vi "Build_Header_String_Array.vi"(0 "ERD Name Array In":string[](array[string]), 1 "ERD Number Array In":string[](array[string]), 2 "ERD Name List":string[](array[string])=[""], 3 "New Header?":bool, 4 "ERD Number":u16) -> (14 "ERD Name Array Out":string[](array[string]), 15 "ERD Number Array Out":string[](array[string]))   [LabVIEW 2021]
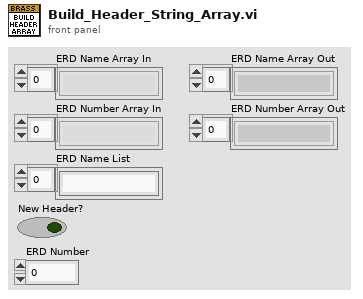
[diagram p1: front panel]
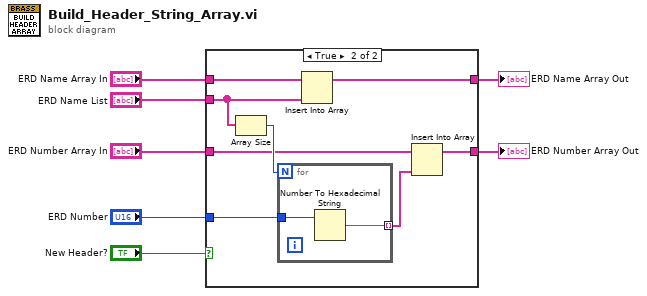
[diagram p0: block diagram]
diagram:
  n1 = case shown="True" "New Header?" {
    tunnel: "ERD Number Array In" -> [w9 w12]
    tunnel: "ERD Number" -> [_ w17]
    tunnel: [w9 w10] -> w4
    tunnel: "ERD Name Array In" -> [w8 w16]
    tunnel: "ERD Name List" -> [_ w13]
    tunnel: [w8 w15] -> w7
    frame False {
    }
    frame True {
      n2 = Array Size(array=w13) -> (size(s)=w14:i32)
      n3 = for {
        N: w14 -> [_]
        tunnel: w17 -> [w19]
        tunnel: [w18] -> w11 mode=indexing
        n4 = Number To Hexadecimal String(2:w19) -> (0:w18:string)  [unwired: 1 in]
      }
      n5 = Insert Into Array(array=w16, new element=w13) -> (w15:string[])  [unwired: 1 in]
      n6 = Insert Into Array(array=w12, new element=w11) -> (w10:string[])  [unwired: 1 in]
    }
  }
  "ERD Name Array Out" <- w7
  "ERD Number Array Out" <- w4
